vi "CloseSysClk.vi"(8 "error in (no error)":errorcluster, 11 "PXI_MultiTrig in":refnum<class "PXI_MultiTrig.lvclass">) -> (0 "error out":errorcluster, 3 "PXI_MultiTrig out":refnum<class "PXI_MultiTrig.lvclass">)   [LabVIEW 2018, in "SyncPlugins.lvlib" / "PXI_MultiTrig.lvclass"]
uses:
  PXI_MultiTrig.lvclass
  PXI_MultiTrig.lvclass/PXI_MultiTrig.ctl
  Accessors/Read SyncWindowsClock.vi
  Accessors/Read SysHandle.vi
  Accessors/Read SysRef.vi
  <vilib>/nisyscfg/Close (System).vi
  <vilib>/nisyscfg/Close (Hardware).vi
  <vilib>/nisyscfg/nisyscfg.lvlib
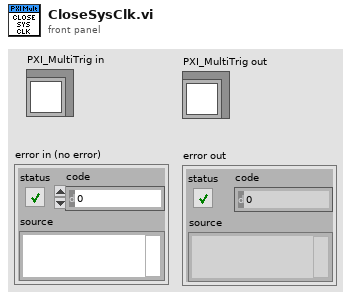
[diagram p1: front panel]
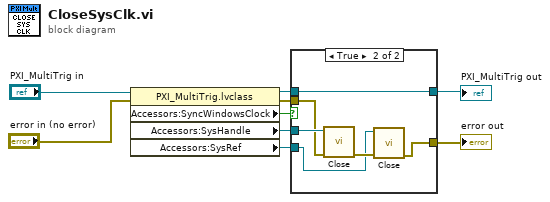
[diagram p0: block diagram]
diagram:
  n1 = property class="PXI_MultiTrig.lvclass"(reference="PXI_MultiTrig in", error in="error in (no error)") -> (reference out=w3:refnum<class "PXI_MultiTrig.lvclass">, error out=w7:errorcluster, "Accessors:SyncWindowsClock"=w6:bool, "Accessors:SysHandle"=w5:refnum<k21>, "Accessors:SysRef"=w1:refnum<k20>)
  n2 = case shown="True" w6 {
    tunnel: w7 -> [w10 w16]
    tunnel: w5 -> [_ w17]
    tunnel: [w10 w13] -> w4
    tunnel: w3 -> [w11 w15]
    tunnel: [w11 w15] -> w2
    tunnel: w1 -> [_ w12]
    frame False {
    }
    frame True {
      n3 = call-poly <vilib>:"Close.vi"("error in (no error)"=w16, "Session in"=w17) -> ("error out"=w14:errorcluster)  [unwired: 9 in]
      n4 = call-poly <vilib>:"Close.vi"("error in (no error)"=w14, "Resource in"=w12) -> ("error out"=w13:errorcluster)  [unwired: 9 in]
    }
  }
  "error out" <- w4
  "PXI_MultiTrig out" <- w2
